vi "DialogBoxSubVI.vi"(10 "Prompt":string) -> (3 "Boolean":bool)   [LabVIEW 2015]
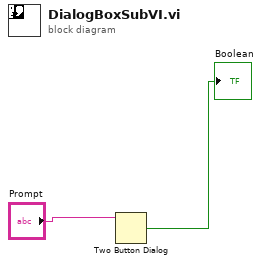
[diagram p0: block diagram]
diagram:
  n1 = Two Button Dialog(message="Prompt") -> (T button?=→"Boolean":bool)  [unwired: 2 in]
